vi "Test_LaunchAndCloseAbstractFramework_NoError.vi"(8 "error in (no error)":errorcluster, 11 "TestCase in":refnum<class "TestIViewModel.lvclass">) -> (0 "error out":errorcluster, 3 "TestCase out":refnum<class "TestIViewModel.lvclass">)   [LabVIEW 2017, in "TestIViewModel.lvclass"]
uses:
  TestIViewModel.lvclass
  Framework/IViewModel/IViewModel/IViewModel.lvclass
  C:/Git/mva-framework/Framework/IViewManager/IViewManager/IViewManager.lvclass
  C:/Program Files (x86)/National Instruments/LabVIEW 2017/vi.lib/ActorFramework/Actor/Actor.lvclass
  Framework/IViewable/IViewable/IViewable.lvclass
  Framework/IModel/IModel/IModel.lvclass
  Framework/IMediator/IMediator/IMediator.lvclass
  Framework/IViewModel/IViewModel/IViewModel.lvclass/IViewModel.ctl
  Framework/IViewManager/IViewManager Messages/Launch Nested Views Msg/Launch Nested Views Msg.lvclass/Launch Nested Views Msg.ctl
  Framework/IViewManager/IViewManager/IViewManager.lvclass/IViewManager.ctl
  <vilib>/ActorFramework/Message Enqueuer/Message Enqueuer.lvclass/Message Enqueuer.ctl
  Framework/IViewManager/IViewManager Messages/Launch Nested Views Msg/Pack Launch Nested Views Msg.vi
  Framework/IViewManager/IViewManager/Write Startup Launch Nested Views Msg.vi
  <vilib>/ActorFramework/Message Enqueuer/Enqueue.vi
  <vilib>/ActorFramework/Stop Msg/Stop Msg.lvclass
  C:/Program Files (x86)/National Instruments/LabVIEW 2017/vi.lib/ActorFramework/Message/Message.lvclass
  <vilib>/ActorFramework/Message Priority Queue/Priority Enqueue.vi
  Framework/IViewable/IApplicationStyle/IApplicationStyle.lvclass
  Framework/IViewManager/IViewManager Messages/Launch Nested Views Msg/Launch Nested Views Msg.lvclass
  <vilib>/ActorFramework/Actor/Actor.lvclass
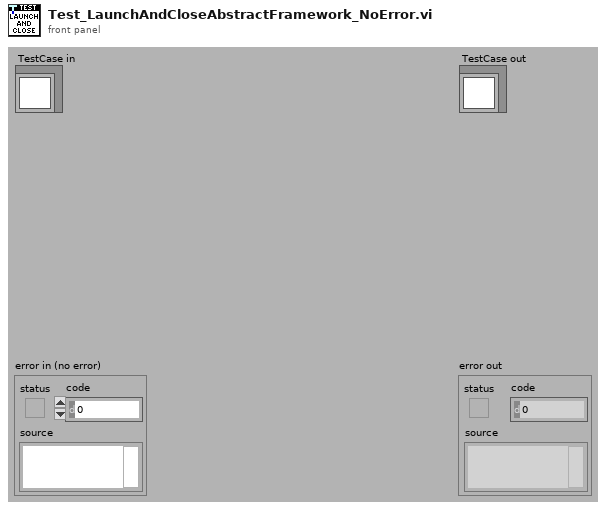
[diagram p1: front panel]
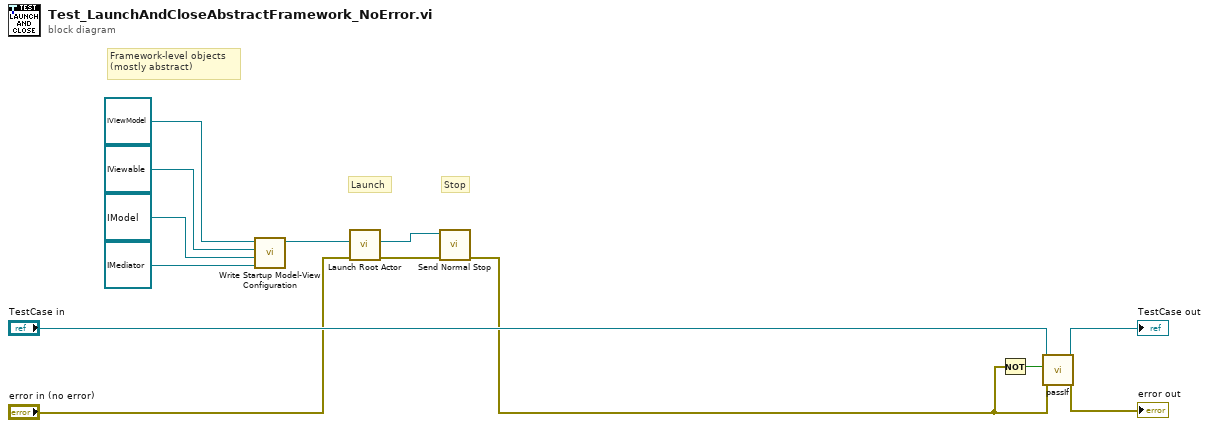
[diagram p0: block diagram]
diagram:
  # "Stop"
  # "Launch"
  # "Framework-level objects\n(mostly abstract)"
  n1 = call "Write Startup Model-View Configuration.vi"("Mediator Type"=refnum<class "IMediator.lvclass"> refnum ("Mediator"), "Model Type"=refnum<class "IModel.lvclass"> refnum ("Model"), "Startup View Configuration"=refnum<class "IViewable.lvclass"> refnum, "IViewModel In"=refnum<class "IViewModel.lvclass"> refnum) -> ("IViewModel Out"=w5:refnum<class "IViewModel.lvclass">)  [unwired: 7 in]
  n2 = call <vilib>:"Launch Root Actor.vi"("error in (no error)"="error in (no error)", "Actor"=w5) -> ("error out"=w3:errorcluster, "Actor's Enqueuer"=w4:refnum<class "Message Enqueuer.lvclass">)  [unwired: 8 in]
  n3 = call <vilib>:"Send Normal Stop.vi"("error in (no error)"=w3, "Message Enqueuer"=w4) -> ("error out"=w1:errorcluster)  [unwired: 9 in]
  n4 = Not(x=w1) -> (.not. x?=w10:bool)
  n5 = call-dynamic "passIf.vi"("error in (no error)"=w1, "pass"=w10, "TestCase in"="TestCase in") -> ("error out"=→"error out":errorcluster, "TestCase out"=→"TestCase out":refnum<class "TestIViewModel.lvclass">)  [unwired: 7 in]
